vi "Word_Set_Selection_Font.vi"(0 "selection in":refnum<k7>, 2 "font":T1 {"font size" format="%.2f"; "strike through" items=["Unchanged", "Yes", "No"]; "underline" items=["Unchanged", "Yes", "No"]; "italic" items=["Unchanged", "Yes", "No"]; "bold" items=["Unchanged", "Yes", "No"]}, 3 "error in":errorcluster) -> (6 "selection out":refnum<k7>, 9 "error out":errorcluster)   [LabVIEW 2017, in "NI_ReportGenerationToolkit.lvlib"]
uses:
  <vilib>/addons/_office/NI_ReportGenerationToolkit.lvlib
  <vilib>/addons/_office/_exclsub.llb/font.ctl
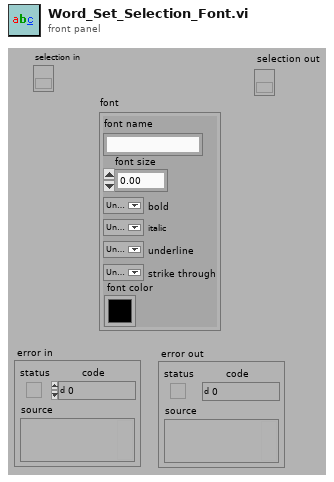
[diagram p1: front panel]
types:
  T1 = typedef "NI_ReportGenerationToolkit.lvlib/font.ctl" = cluster{"font name":string, "font size":dbl, "bold":u16, "italic":u16, "underline":u16, "strike through":u16, "font color":u32}
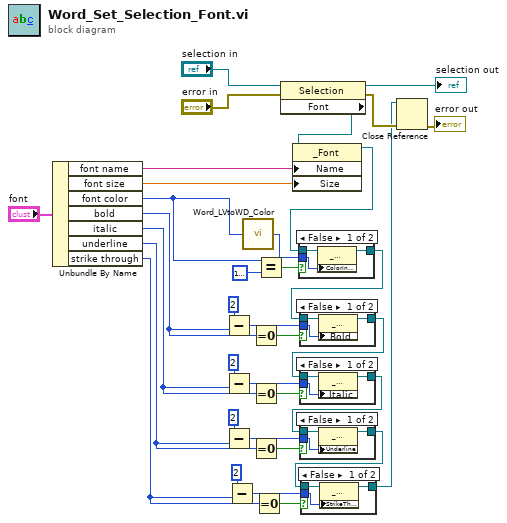
[diagram p0: block diagram]
diagram:
  n1 = Unbundle By Name("font") -> ("font name"=w30:string, "font size"=w29:dbl, "font color"=w1:u32, "bold"=w25:u16, "italic"=w15:u16, "underline"=w14:u16, "strike through"=w13:u16)
  n2 = Subtract(x=2, y=w25) -> (x-y=w26:i32)
  n3 = Subtract(x=2, y=w15) -> (x-y=w24:i32)
  n4 = Subtract(x=2, y=w14) -> (x-y=w19:i32)
  n5 = Subtract(x=2, y=w13) -> (x-y=w18:i32)
  n6 = call <vilib>:"Word_LVtoWD_Color.vi"("LabVIEW color"=w1) -> ("word color table index"=w3:i32)
  n7 = Equal To 0?(x=w25) -> (x = 0?=w28:bool)
  n8 = Equal To 0?(x=w15) -> (x = 0?=w22:bool)
  n9 = Equal To 0?(x=w14) -> (x = 0?=w21:bool)
  n10 = Equal To 0?(x=w13) -> (x = 0?=w16:bool)
  n11 = Equal?(x=w1, y=u32 16777216) -> (x = y?=w9:bool)
  n12 = property class="Selection"(reference="selection in", error in="error in") -> (reference out=→"selection out":refnum<k7>, error out=w32:errorcluster, "Font"=w5:refnum<k7>)
  n13 = property class="_Font"(reference=w5, "Name"=w30, "Size"=w29) -> (reference out=w8:refnum<k7>)  [unwired: 1 in, 1 out]
  n14 = case shown="False" w9 {
    tunnel: w8 -> [w38 w39]
    tunnel: w3 -> [w37 _]
    tunnel: [w36 w39] -> w7
    frame False {
      n15 = property class="_Font"(reference=w38, "ColorIndex"=w37) -> (reference out=w36:refnum<k7>)  [unwired: 1 in, 1 out]
    }
    frame True {
    }
  }
  n16 = case shown="False" w28 {
    tunnel: w7 -> [w42 w43]
    tunnel: w26 -> [w41 _]
    tunnel: [w40 w43] -> w12
    frame False {
      n17 = property class="_Font"(reference=w42, "Bold"=w41) -> (reference out=w40:refnum<k7>)  [unwired: 1 in, 1 out]
    }
    frame True {
    }
  }
  n18 = case shown="False" w22 {
    tunnel: w12 -> [w46 w47]
    tunnel: w24 -> [w45 _]
    tunnel: [w44 w47] -> w11
    frame False {
      n19 = property class="_Font"(reference=w46, "Italic"=w45) -> (reference out=w44:refnum<k7>)  [unwired: 1 in, 1 out]
    }
    frame True {
    }
  }
  n20 = case shown="False" w21 {
    tunnel: w11 -> [w50 w51]
    tunnel: w19 -> [w49 _]
    tunnel: [w48 w51] -> w10
    frame False {
      n21 = property class="_Font"(reference=w50, "Underline"=w49) -> (reference out=w48:refnum<k7>)  [unwired: 1 in, 1 out]
    }
    frame True {
    }
  }
  n22 = case shown="False" w16 {
    tunnel: w10 -> [w54 w55]
    tunnel: w18 -> [w53 _]
    tunnel: [w52 w55] -> w4
    frame False {
      n23 = property class="_Font"(reference=w54, "StrikeThrough"=w53) -> (reference out=w52:refnum<k7>)  [unwired: 1 in, 1 out]
    }
    frame True {
    }
  }
  n24 = Close Reference(reference=w4, error in (no error)=w32) -> (error out=→"error out":errorcluster)
